vi "Test Set Cell Value 2D Array String.vi"(11 "Test Case In":refnum<class "Test Open Xml.lvclass">) -> (0 "error out":errorcluster, 3 "Test Case Out":refnum<class "Test Open Xml.lvclass">)   [LabVIEW 2025, in "Test Open Xml.lvclass"]
uses:
  Test Open Xml.lvclass
  C:/Program Files/National Instruments/LabVIEW 2025/vi.lib/Astemes/LUnit/Test Case.lvclass
  <vilib>/Astemes/LUnit/Test Case.lvclass/Test Case.ctl
  f76079c9-ef62-41ac-a871-70fbb9772100.vi
  f76079c9-ef62-41ac-a871-70fbb9772100.vi/379da758-ac74-47b7-b442-37c8af95aa11.vi
  Source/Excel Cell Address to Numeric Indices.vi
  Source/Numeric Indices to Excel Cell Address.vi
  <vilib>/Astemes/LUnit/Append Fail Result.vi
  <vilib>/Astemes/LUnit/Append Pass Result.vi
  <vilib>/Astemes/LUnit/Run In UI.vi
  <vilib>/Utility/error.llb/Clear Errors.vi
  Source/Get WorksheetPart.vi
  Source/Get or Add Cell.vi
  Source/Create CellValue.vi
  Source/Set CellValue.vi
  Source/Set Cell DataType.vi
  <vilib>/Astemes/LUnit/Test Case.lvclass
  Source/Open Xml.lvlib
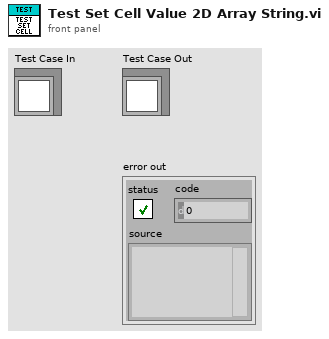
[diagram p1: front panel]
types:
  T1 = typedef "Open Xml.lvlib/Cell DataType.ctl" = enum16{"Void", "Boolean", "Number", "Error", "SharedString", "String", "InlineString", "Date"}
  T2 = cluster{"Number":dbl, "String":string, "Boolean":bool, "Time Stamp":timestamp, "Error":errorcluster}[][]
  T3 = enum16{"Void", "Boolean", "Number", "Error", "SharedString", "String", "InlineString", "Date"}
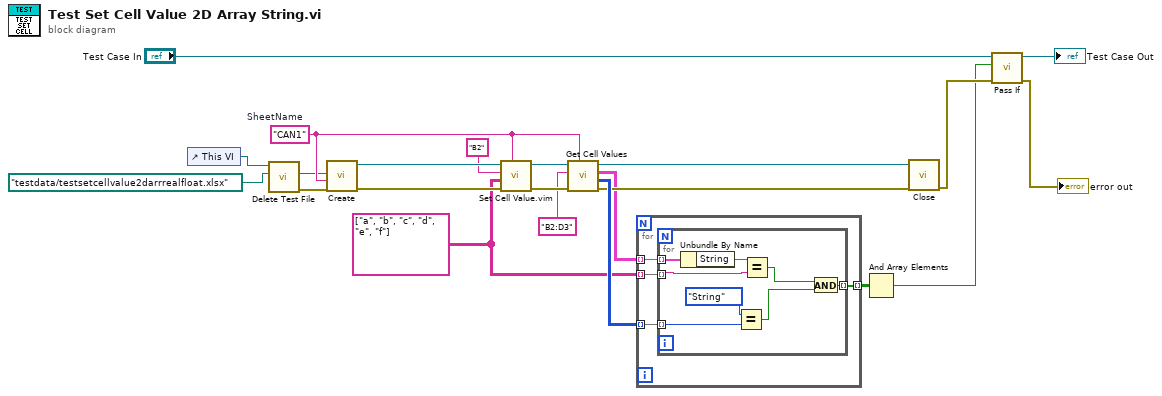
[diagram p0: block diagram]
diagram:
  w4 = string[][] [["a", "b", "c"], ["d", "e", "f"]]
  w15 = "CAN1"  # SheetName
  n1 = control-ref of="This VI"() -> (w14:refnum<vi>)
  n2 = call "Delete Test File.vi"("name or relative path"=path "testdata/testsetcellvalue2darrrealfloat.xlsx", "VI in"=w14) -> ("error out"=w12:errorcluster, "deleted path"=w11:path)  [unwired: 8 in]
  n3 = call "Create.vi"("error in"=w12, "SheetName"=w15, "Path"=w11) -> ("error out"=w18:errorcluster, "SpreadsheetDoc"=w19:refnum<k24>)  [unwired: 7 in]
  n4 = call "Set Cell Value.vim"("Sheet Name"=w15, "error in"=w18, "Value"=w4, "Cell Address"="B2", "SpreadsheetDoc in"=w19) -> ("error out"=w10:errorcluster, "SpreadsheetDoc out"=w9:refnum<k24>)  [unwired: 5 in]
  n5 = call "Get Cell Values.vi"("Sheet Name"=w15, "error in"=w10, "Cell Addresses"="B2:D3", "SpreadsheetDoc in"=w9) -> ("error out"=w5:errorcluster, "Types"=w8:T1[][], "Cell Values"=w3:T2, "SpreadsheetDoc out"=w16:refnum<k24>)  [unwired: 4 in]
  n6 = for {
    tunnel: w8 -> [w26] mode=indexing
    tunnel: w4 -> [w25] mode=indexing
    tunnel: w3 -> [w24] mode=indexing
    tunnel: [w23] -> w2 mode=indexing
    n7 = for {
      tunnel: w26 -> [w33] mode=indexing
      tunnel: w25 -> [w28] mode=indexing
      tunnel: w24 -> [w31] mode=indexing
      tunnel: [w30] -> w23 mode=indexing
      n8 = Unbundle By Name(w31) -> ("String"=w29:string)
      n9 = Equal?(x=T3."String", y=w33) -> (x = y?=w32:bool)
      n10 = Equal?(x=w29, y=w28) -> (x = y?=w27:bool)
      n11 = And(x=w27, y=w32) -> (x .and. y?=w30:bool)
    }
  }
  n12 = And Array Elements(Boolean array=w2) -> (logical AND=w1:bool)
  n13 = call "Close.vi"("error in"=w5, "SpreadsheetDoc"=w16) -> ("error out"=w17:errorcluster)  [unwired: 9 in]
  n14 = call <vilib>:"Pass If.vi"("error in (no error)"=w17, "Pass?"=w1, "LUnit Test Case In"="Test Case In") -> ("error out"=→"error out":errorcluster, "LUnit Test Case Out"=→"Test Case Out":refnum<class "Test Open Xml.lvclass">)  [unwired: 7 in]
